vi "SaveData.vi"(4 "Name Rings?":bool, 5 "Location":u16(ring) items=["RRI", "Hawaii"], 6 "Sector Angle":i32(slide)=360 min=0 max=360 step=45 scale=0.0..360.0, 7 "Scan Data":i16[][][][](array[numeric]), 8 "#Trans Rings":i8=5, 9 "1-D Scan?":bool, 10 "Array":T1(array[cluster]) {"Scan Settings"."prf (kHz)" format="%.2f"; "Scan Settings"."GAIN(db)" items=["26.0", "40.0", "54.0"]; "Scan Settings"."LP FILT(IN MHz)" items=["20", "50", "100", "200"]; "Scan Settings"."HP FILT(IN KHz)" items=["1", "1000", "3000", "10000"]; "Scan Settings"."DAMPING (IN Ohm)" items=["7", "10", "16", "20", "26", "30", "40", "50"]; "Scan Settings"."ENERGY(UJ)" items=["1", "2", "4", "8", "16", "32"]; "Therapy Parameters"."Therapy amplitude (mV)" format="%.2f"; "Therapy Parameters"."Time on" format="%.2f"; "Therapy Parameters"."Theraputic Freq (MHz)" format="%.2f"; "Digitizer delay\n (ms)" format="%.2f"; "avg num" format="%.2f"}, 11 "Type of scan":u16(ring) items=["Therapy with scan", "M scan", "M scan w/ therapy", "1-D B Scan", "1-D B Scan w/ Therapy", "2-D B Scan", "2-D B Scan w/ Therapy", "Rotational Scan"]) -> ()   [LabVIEW 2022 SP3]
uses:
  ScanningControl/Motion Controllers/-MotionRoutines/MotionGlobals.vi
panel:
  in  "Case Constant\n(See Context Help)":bool=TRUE
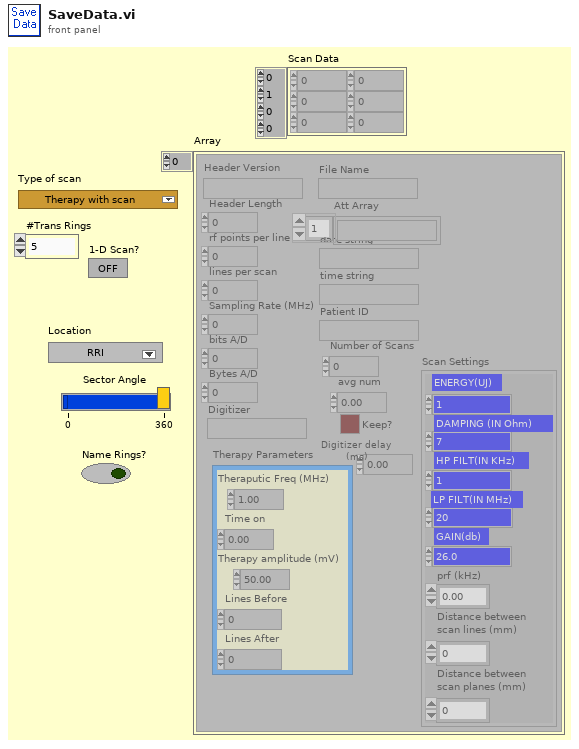
[diagram p1: front panel]
types:
  T1 = cluster{"Header Version":string, "Header Length":i32, "rf points per line":u16, "lines per scan":u16, "Sampling Rate (MHz)":i32, "bits A/D":i32, "Bytes A/D":i32, "Digitizer":string, "File Name":string, "Att Array":string[], "date string":string, "time string":string, "Patient ID":string, "Number of Scans":i32, "avg num":dbl, "Keep?":bool, "Digitizer delay\n (ms) ":dbl, "Therapy Parameters":cluster{"Theraputic Freq (MHz)":sgl, "Time on":sgl, "Therapy amplitude (mV)":sgl, "Lines Before":u16, "Lines After":u16}, "Scan Settings":cluster{"ENERGY(UJ)":u8, "DAMPING (IN Ohm)":u8, "HP FILT(IN KHz) ":u8, "LP FILT(IN MHz)":u8, "GAIN(db)":u8, "prf (kHz)":sgl, "Distance between\nscan lines (mm)":u16, "Distance between\nscan planes (mm)":u16}}[]
  T2 = cluster{"Therapy frequency (MHz)":dbl, dbl, "Therapy amplitude (mV)":dbl, i32, i32}
  T3 = cluster{"header info":cluster{"Header":string, "Head length":i16}, "A/D info":cluster{"# rf points per line":u16, "# lines per scan":u16, "sample rate MHz":u16, "# A/D bits":i16, "# bytes per A/D":u16, "TGC Flag":u16, "A/D Type":string}, "Tranducer Info":cluster{"bandwidth":sgl, "center freq":sgl, "start freq":sgl, "ID":i32}, "Scan Info":cluster{"delay":sgl, "pivot distance":sgl, "sector scan angle":sgl, "operator":string, "Scan Mode":string, "location":string}, "Time/Date Info":cluster{"date":string, "time":string}, "RF Info":cluster{"RF file name":string, "RF file att":string, "RF cal file name":string, "RF cal file att":string}, "Patient Info":cluster{"ID":string, "extended ID":string, "age":u16, "sex":string, "previously\nscanned":string, "bandwidth":sgl, "age 2":u8, "age 3":u16, "Distance between\nscan planes (mm) 2":u16}, "Tissue Type":cluster{"organ":i16, "disease type":i16, "disease location":i16}, "Calibration Info":cluster{"flag":i16, "offset of spectrum":i32}, "Comment":string, "Misc Params":cluster{"avg num":i16, "c speed":i16, "DivdeBy":i16}, "Therapy Parameters":cluster{"Theraputic Freq (MHz)":sgl, "Time on (s)":sgl, "Therapy amplitude (mV)":sgl, "Lines Before":u16, "Lines After":u16}, "Scan Settings":cluster{"Energy (microJ)":u8, "Damping (In Ohm)":u8, "HP Filt(KHz)":u8, "LP Filt (MHz)":u8, "Gain (db)":u8, "prf (kHz)":sgl, "Distance between\nscan lines (mm)":u16, "Distance between\nscan planes (mm)":u16}}
  T4 = cluster{"Header Version":string, "Header Length":i32, "rf points per line":u16, "lines per scan":u16, "Sampling Rate (MHz)":i32, "bits A/D":i32, "Bytes A/D":i32, "Digitizer":string, "File Name":string, "Att Array":string[], "date string":string, "time string":string, "Patient ID":string, "Number of Scans":i32, "avg num":dbl, "Keep?":bool, "Digitizer delay\n (ms) ":dbl, "Therapy Parameters":cluster{"Theraputic Freq (MHz)":sgl, "Time on":sgl, "Therapy amplitude (mV)":sgl, "Lines Before":u16, "Lines After":u16}, "Scan Settings":cluster{"ENERGY(UJ)":u8, "DAMPING (IN Ohm)":u8, "HP FILT(IN KHz) ":u8, "LP FILT(IN MHz)":u8, "GAIN(db)":u8, "prf (kHz)":sgl, "Distance between\nscan lines (mm)":u16, "Distance between\nscan planes (mm)":u16}}
  T5 = cluster{"Theraputic Freq (MHz)":sgl, "Time on":sgl, "Therapy amplitude (mV)":sgl, "Lines Before":u16, "Lines After":u16}
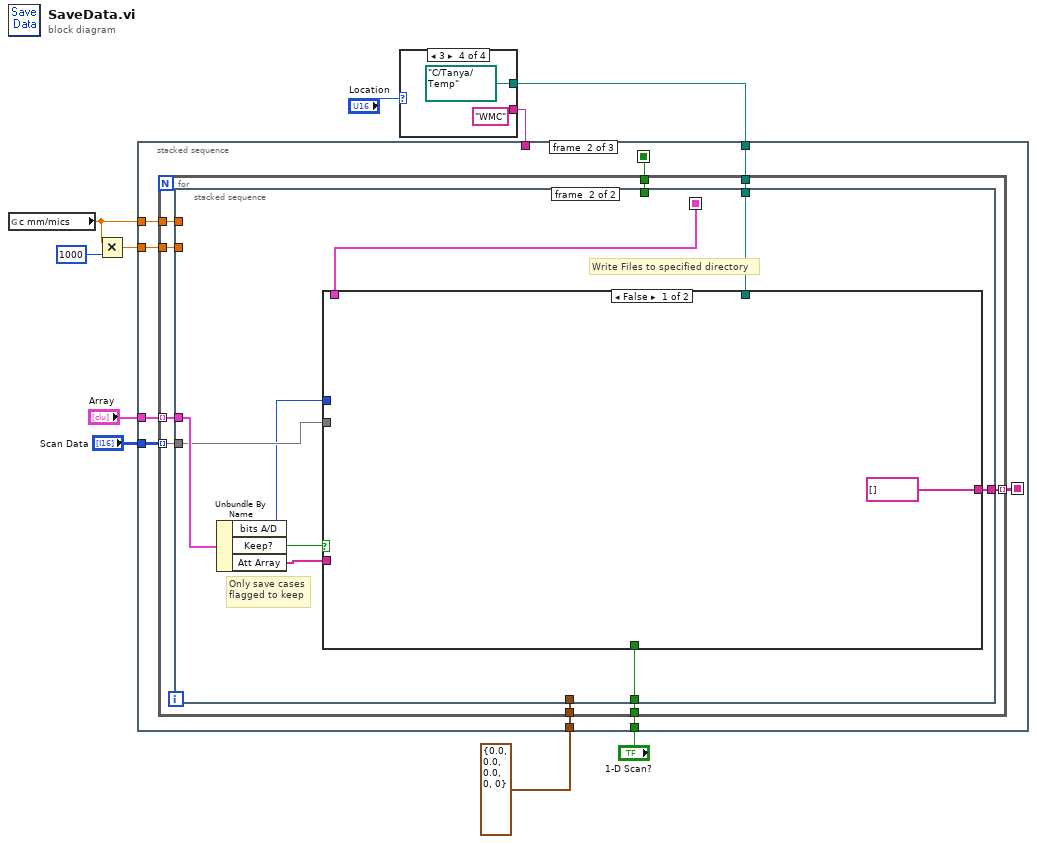
[diagram p0: block diagram]
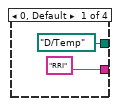
[diagram p2: hidden frame]
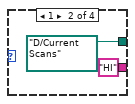
[diagram p3: hidden frame]
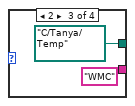
[diagram p4: hidden frame]
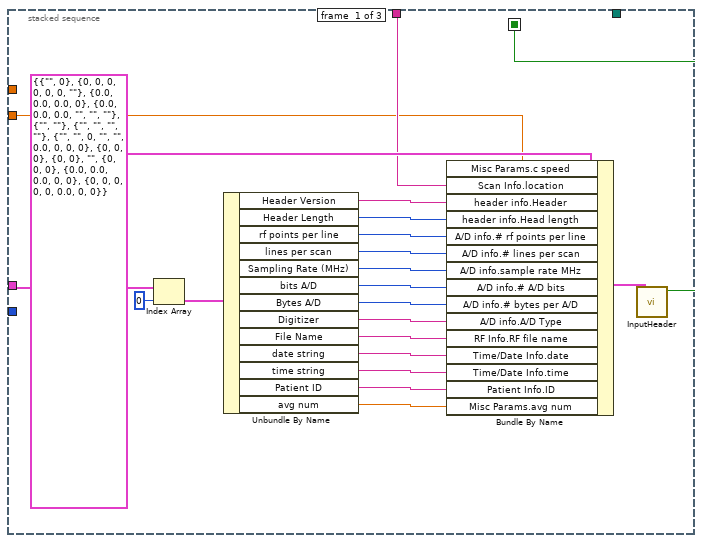
[diagram p5: hidden frame]
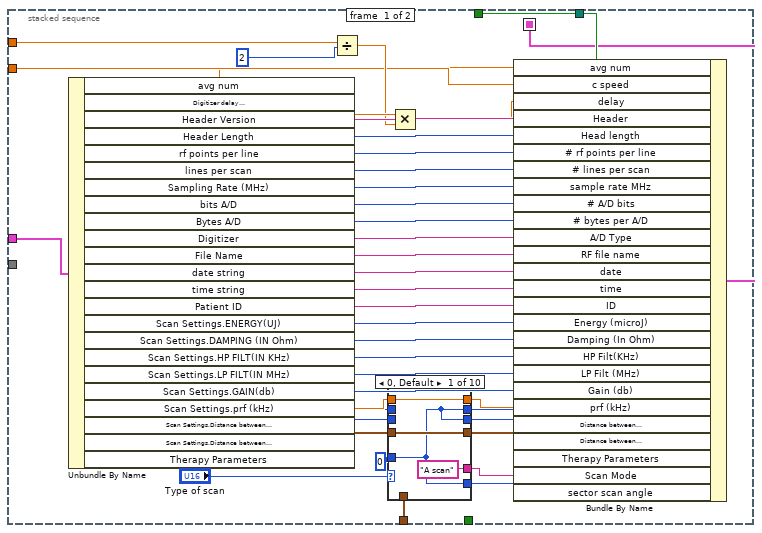
[diagram p6: hidden frame]
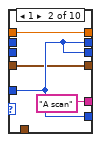
[diagram p7: hidden frame]
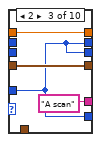
[diagram p8: hidden frame]
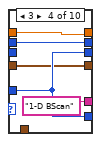
[diagram p9: hidden frame]
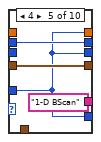
[diagram p10: hidden frame]
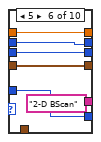
[diagram p11: hidden frame]
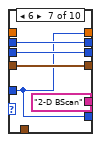
[diagram p12: hidden frame]
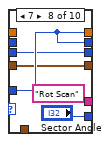
[diagram p13: hidden frame]
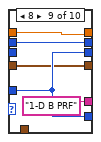
[diagram p14: hidden frame]
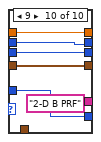
[diagram p15: hidden frame]
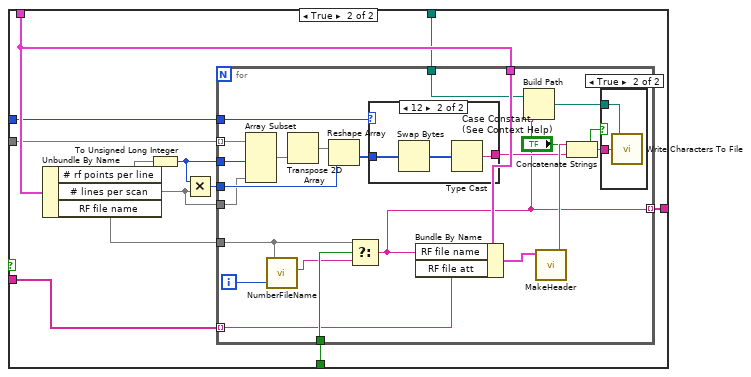
[diagram p16: hidden frame]
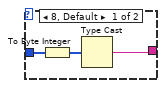
[diagram p17: hidden frame]
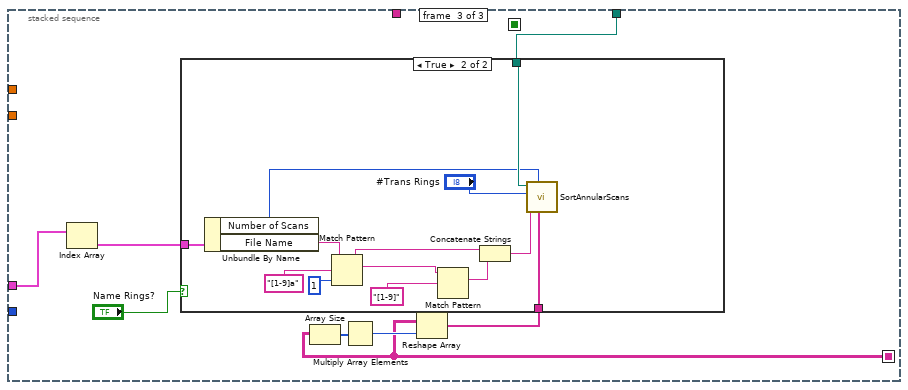
[diagram p19: hidden frame]
diagram:
  n1 = global read "MotionGlobals.vi" "c mm/mics"() -> (w3:sgl)
  n2 = Multiply(x=w3, y=1000) -> (x*y=w1:sgl)
  n3 = case shown="3" "Location" {
    tunnel: ["RRI" "HI" "WMC" "WMC"] -> w7
    tunnel: [path "D:/Temp" path "D:/Current Scans" path "C:/Tanya/Temp" path "C:/Tanya/Temp"] -> w6
    frame 0, Default {
    }
    frame 1 {
    }
    frame 2 {
    }
    frame 3 {
    }
  }
  n4 = stacked-sequence {
    seq-local: [w23 _ _] -> [_ w45 _]
    seq-local: [_ w43 _] -> [_ _ w199]
    tunnel: "Array" -> [w27 w48 w204]
    tunnel: "1-D Scan?" -> [_ w47 _]
    tunnel: w6 -> [_ w46 w205]
    tunnel: T2 {"Therapy frequency (MHz)"=0.0, 0.0, "Therapy amplitude (mV)"=0.0, 0, 0} ("Output Cluster") -> [_ w44 _]
    tunnel: w7 -> [w21 _ _]
    tunnel: "Scan Data" -> [_ w42 _]
    tunnel: w3 -> [_ w41 _]
    tunnel: w1 -> [w19 w40 _]
    frame #0 {
      n5 = Index Array(array=w27, index=0 ("Index")) -> (element=w25:T4)
      n6 = Unbundle By Name(w25) -> ("Header Version"=w38:string, "Header Length"=w39:i32, "rf points per line"=w37:u16, "lines per scan"=w36:u16, "Sampling Rate (MHz)"=w35:i32, "bits A/D"=w34:i32, "Bytes A/D"=w33:i32, "Digitizer"=w32:string, "File Name"=w31:string, "date string"=w30:string, "time string"=w29:string, "Patient ID"=w28:string, "avg num"=w20:dbl)
      n7 = Bundle By Name(cluster=T3 {"header info"={"Header"="", "Head length"=0}, "A/D info"={"# rf points per line"=0, "# lines per scan"=0, "sample rate MHz"=0, "# A/D bits"=0, "# bytes per A/D"=0, "TGC Flag"=0, "A/D Type"=""}, "Tranducer Info"={"bandwidth"=0.0, "center freq"=0.0, "start freq"=0.0, "ID"=0}, "Scan Info"={"delay"=0.0, "pivot distance"=0.0, "sector scan angle"=0.0, "operator"="", "Scan Mode"="", "location"=""}, "Time/Date Info"={"date"="", "time"=""}, "RF Info"={"RF file name"="", "RF file att"="", "RF cal file name"="", "RF cal file att"=""}, "Patient Info"={"ID"="", "extended ID"="", "age"=0, "sex"="", "previously\nscanned"="", "bandwidth"=0.0, "age 2"=0, "age 3"=0, "Distance between\nscan planes (mm) 2"=0}, "Tissue Type"={"organ"=0, "disease type"=0, "disease location"=0}, "Calibration Info"={"flag"=0, "offset of spectrum"=0}, "Comment"="", "Misc Params"={"avg num"=0, "c speed"=0, "DivdeBy"=0}, "Therapy Parameters"={"Theraputic Freq (MHz)"=0.0, "Time on (s)"=0.0, "Therapy amplitude (mV)"=0.0, "Lines Before"=0, "Lines After"=0}, "Scan Settings"={"Energy (microJ)"=0, "Damping (In Ohm)"=0, "HP Filt(KHz)"=0, "LP Filt (MHz)"=0, "Gain (db)"=0, "prf (kHz)"=0.0, "Distance between\nscan lines (mm)"=0, "Distance between\nscan planes (mm)"=0}} ("Output Element"), "Misc Params.c speed"=w19, "Scan Info.location"=w21, "header info.Header"=w38, "header info.Head length"=w39, "A/D info.# rf points per line"=w37, "A/D info.# lines per scan"=w36, "A/D info.sample rate MHz"=w35, "A/D info.# A/D bits"=w34, "A/D info.# bytes per A/D"=w33, "A/D info.A/D Type"=w32, "RF Info.RF file name"=w31, "Time/Date Info.date"=w30, "Time/Date Info.time"=w29, "Patient Info.ID"=w28, "Misc Params.avg num"=w20) -> (w24:T3)
      n8 = call "InputHeader.vi"("Save Path"=w24) -> ("Empty String?"=w23:bool)  [unwired: 3 in, 3 out]
    }
    frame #1 {
      n9 = for {
        tunnel: w48 -> [w57] mode=indexing
        tunnel: w46 -> [w56]
        tunnel: w47 -> [w55]
        tunnel: w45 -> [w54]
        tunnel: w44 -> [w53]
        tunnel: [w52] -> w43 mode=indexing
        tunnel: w42 -> [w51] mode=indexing
        tunnel: w41 -> [w50]
        tunnel: w40 -> [w49]
        n10 = stacked-sequence {
          seq-local: [w76 _] -> [_ w154]
          tunnel: w57 -> [w86 w151]
          tunnel: w56 -> [_ w153]
          tunnel: w55 -> [_ w152]
          tunnel: w54 -> [w82 _]
          tunnel: w53 -> [w65 _]
          tunnel: [_ w149] -> w52
          tunnel: w51 -> [_ w147]
          tunnel: w50 -> [w60 _]
          tunnel: w49 -> [w59 _]
          frame #0 {
            n11 = Unbundle By Name(w86) -> ("avg num"=w58:dbl, "Digitizer delay\n (ms)"=w84:dbl, "Header Version"=w96:string, "Header Length"=w97:i32, "rf points per line"=w95:u16, "lines per scan"=w94:u16, "Sampling Rate (MHz)"=w93:i32, "bits A/D"=w92:i32, "Bytes A/D"=w91:i32, "Digitizer"=w90:string, "File Name"=w89:string, "date string"=w88:string, "time string"=w87:string, "Patient ID"=w85:string, "Scan Settings.ENERGY(UJ)"=w80:u8, "Scan Settings.DAMPING (IN Ohm)"=w81:u8, "Scan Settings.HP FILT(IN KHz)"=w79:u8, "Scan Settings.LP FILT(IN MHz)"=w78:u8, "Scan Settings.GAIN(db)"=w77:u8, "Scan Settings.prf (kHz)"=w75:sgl, "Scan Settings.Distance between\nscan lines (mm)"=w71:u16, "Scan Settings.Distance between\nscan planes (mm)"=w70:u16, "Therapy Parameters"=w67:T5)
            n12 = Divide(x=w60, y=2) -> (x/y=w61:sgl)
            n13 = case shown="0, Default" "Type of scan" {
              tunnel: ["A scan" "A scan" "A scan" "1-D BScan" "1-D BScan" "2-D BScan" "2-D BScan" "Rot Scan" "1-D B PRF" "2-D B PRF"] -> w68
              tunnel: [w100 w104 w108 w111 w115 w120 w125 w134 w136 w141] -> w63
              tunnel: w75 -> [w100 w104 w108 w111 _ w120 _ _ w136 w141]
              tunnel: u16 0 -> [w98 w103 w106 w112 w115 w121 w125 w134 w137 w142]
              tunnel: [w98 w103 w106 w113 w117 w123 w127 w134 w138 w144] -> w73
              tunnel: [w98 w103 w106 w112 w115 w122 w128 w133 w137 w143] -> w72
              tunnel: w71 -> [_ _ _ w113 w117 w123 w127 _ w138 w144]
              tunnel: w70 -> [_ _ _ _ _ w122 w128 w133 _ w143]
              tunnel: [w99 w102 w107 w110 w116 w119 w126 w132 w135 w140] -> w66
              tunnel: w67 -> [w99 w102 w107 w110 w116 w119 w126 w132 w135 w140]
              tunnel: w65 -> [_ _ _ _ _ _ _ _ _ _]
              tunnel: [w98 w103 w106 w112 w115 w121 w125 "Sector Angle" w137 w142] -> w64
              frame 0, Default {
              }
              frame 1 {
              }
              frame 2 {
              }
              frame 3 {
              }
              frame 4 {
              }
              frame 5 {
              }
              frame 6 {
              }
              frame 7 {
              }
              frame 8 {
              }
              frame 9 {
              }
            }
            n14 = Multiply(x=w84, y=w61) -> (x*y=w83:dbl)
            n15 = Bundle By Name(cluster=w82, "avg num"=w58, "c speed"=w59, "delay"=w83, "Header"=w96, "Head length"=w97, "# rf points per line"=w95, "# lines per scan"=w94, "sample rate MHz"=w93, "# A/D bits"=w92, "# bytes per A/D"=w91, "A/D Type"=w90, "RF file name"=w89, "date"=w88, "time"=w87, "ID"=w85, "Energy (microJ)"=w80, "Damping (In Ohm)"=w81, "HP Filt(KHz)"=w79, "LP Filt (MHz)"=w78, "Gain (db)"=w77, "prf (kHz)"=w63, "Distance between\nscan lines (mm)"=w73, "Distance between\nscan planes (mm)"=w72, "Therapy Parameters"=w66, "Scan Mode"=w68, "sector scan angle"=w64) -> (w76:cluster{})
          }
          frame #1 {
            # "Only save cases\nflagged to keep"
            # "Write Files to specified directory"
            n16 = Unbundle By Name(w151) -> ("bits A/D"=w146:i32, "Keep?"=w150:bool, "Att Array"=w148:string[])
            n17 = case shown="False" w150 {
              tunnel: w154 -> [_ w165]
              tunnel: w153 -> [_ w164]
              tunnel: w152 -> [_ w162]
              tunnel: [string[] [] w161] -> w149
              tunnel: w148 -> [_ w160]
              tunnel: w147 -> [_ w159]
              tunnel: w146 -> [_ w157]
              frame False {
              }
              frame True {
                n18 = Unbundle By Name(w165) -> ("# rf points per line"=w167, "# lines per scan"=w158, "RF file name"=w163)
                n19 = To Unsigned Long Integer(number=w167) -> (unsigned 32bit integer=w156:u32)
                n20 = Multiply(x=w156, y=w158) -> (x*y=w166:u32)
                n21 = for {
                  tunnel: w159 -> [w171] mode=indexing
                  tunnel: w166 -> [w189]
                  tunnel: w165 -> [w187]
                  tunnel: w164 -> [w184]
                  tunnel: w163 -> [w179]
                  tunnel: w162 -> [w180]
                  tunnel: [w175] -> w161 mode=indexing
                  tunnel: w160 -> [w173] mode=indexing
                  tunnel: w157 -> [w172]
                  tunnel: w158 -> [w169]
                  tunnel: w156 -> [w168]
                  i -> [w177]
                  n22 = Array Subset(array=w171, length (row)=w168, length (col)=w169) -> (w170:i16[][])  [unwired: 2 in]
                  n23 = call "NumberFileName.vi"("File number"=w177, "file name"=w179) -> ("Numbered File"=w178:string)  [unwired: 1 in]
                  n24 = Transpose 2D Array(2D array=w170) -> (transposed array=w181:i16[][])
                  n25 = Reshape Array(w181, w189) -> (w188:i16[])
                  n26 = Select(t=w179, s=w180, f=w178) -> (s? t:f=w175:string)
                  n27 = case shown="12" w172 {
                    tunnel: w188 -> [w190 w194]
                    tunnel: [w191 w195] -> w185
                    frame 8, Default {
                      n28 = To Byte Integer(number=w190) -> (8bit integer=w192:i8[])
                      n29 = Type Cast(x=w192) -> (*(type *) &x=w191:string)  [unwired: 1 in]
                    }
                    frame 12 {
                      n30 = Swap Bytes(anything=w194) -> (byte swapped=w193:i16[])
                      n31 = Type Cast(x=w193) -> (*(type *) &x=w195:string)  [unwired: 1 in]
                    }
                  }
                  n32 = Bundle By Name(cluster=w187, "RF file name"=w175, "RF file att"=w173) -> (w176:cluster{})
                  n33 = Build Path(base path=w184, name or relative path=w175) -> (appended path=w183:path)
                  n34 = call "MakeHeader.vi"("Header In"=w176) -> ("Header String"=w186:string)  [unwired: 6 in]
                  n35 = Concatenate Strings(w186, w185) -> (w182:string)
                  n36 = case shown="True" "Case Constant\n(See Context Help)" {
                    tunnel: w183 -> [_ w197]
                    tunnel: w182 -> [_ w196]
                    frame False {
                    }
                    frame True {
                      n37 = call <vilib>:"Write Characters To File.vi"("character string"=w196, "file path (dialog if empty)"=w197) -> ()  [unwired: 3 in, 1 out]
                    }
                  }
                }
              }
            }
          }
        }
      }
    }
    frame #2 {
      n38 = Index Array(array=w204) -> (element=w203:T4)  [unwired: 1 in]
      n39 = Array Size(array=w199) -> (size(s)=w201:i32[])
      n40 = Multiply Array Elements(1:w201) -> (0:w200:i32)
      n41 = Reshape Array(w199, w200) -> (w202:string[])
      n42 = case shown="True" "Name Rings?" {
        tunnel: w205 -> [_ w218]
        tunnel: w203 -> [_ w217]
        tunnel: w202 -> [_ w216]
        frame False {
        }
        frame True {
          n43 = Unbundle By Name(w217) -> ("Number of Scans"=w206:i32, "File Name"=w214:string)
          n44 = Match Pattern(string=w214, regular expression="[1-9]a", offset (0)=1) -> (before substring=w209:string, match substring=w210:string)  [unwired: 2 out]
          n45 = Match Pattern(string=w210, regular expression="[1-9]") -> (match substring=w207:string)  [unwired: 1 in, 3 out]
          n46 = Concatenate Strings(w209, w207) -> (w208:string)
          n47 = call "SortAnnularScans.vi"("file names"=w216, "Scan Planes"=w206, "RootName"=w208, "Transmit Rings"="#Trans Rings", "directory path"=w218) -> ()  [unwired: 3 in]
        }
      }
    }
  }
